vi "Schedule To Operations on Machines.vi"(9 "Number of Jobs":i32, 10 "Number of Machines":i32, 11 "Schedule":u16[](array[numeric])) -> (3 "Operations On Machines":i32[][](array[numeric]))   [LabVIEW 2013, in "GanntChart.lvclass"]
uses:
  GanntChart.lvclass
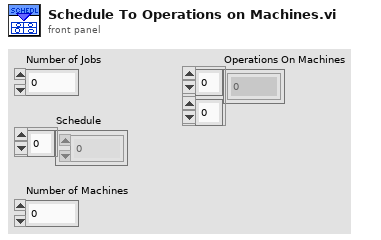
[diagram p1: front panel]
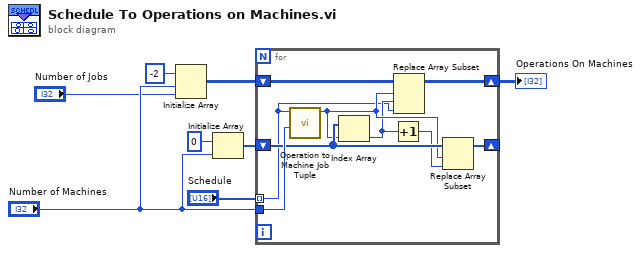
[diagram p0: block diagram]
diagram:
  n1 = Initialize Array(-2, "Number of Machines", "Number of Jobs") -> (w4:i32[][])
  n2 = Initialize Array(0 ("element"), "Number of Machines") -> (w2:i32[])
  n3 = for {
    tunnel: "Schedule" -> [w9] mode=indexing
    tunnel: "Number of Machines" -> [w17]
    shift-right: [w15] -> w1
    shift-left: w4 -> [w16]
    shift-right: [w10] -> _
    shift-left: w2 -> [w14]
    n4 = call "Operation to Machine Job Tuple.vi"("Number of Machines"=w17, "Operation Number"=w9) -> ("Machine No"=w13:i32)  [unwired: 8 in, 1 out]
    n5 = Index Array(array=w14, index=w13) -> (element=w12:i32)
    n6 = Increment(x=w12) -> (x+1=w11:i32)
    n7 = Replace Array Subset(array=w16, new element=w9, index (row)=w13, index (col)=w12) -> (w15:i32[][])
    n8 = Replace Array Subset(array=w14, new element=w11, index=w13) -> (w10:i32[])
  }
  "Operations On Machines" <- w1
